vi "S2C_Access_ReadSettings.vi"(8 "Error In":errorcluster) -> (0 "Error Out":errorcluster)   [LabVIEW 2015]
doc: "Reads the data contained within the Settings file and loads the data into VI specific global variables."
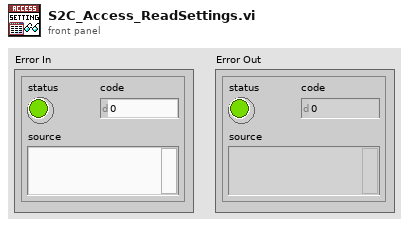
[diagram p1: front panel]
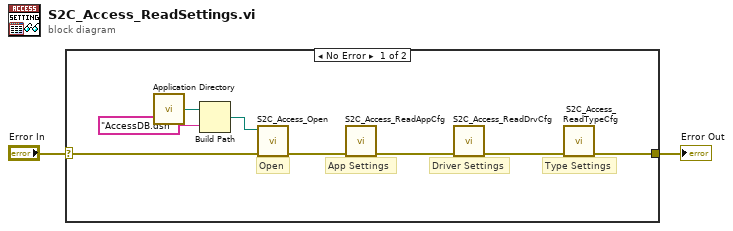
[diagram p0: block diagram]
diagram:
  n1 = case shown="No Error" "Error In" {
    selector: "Error In" -> [w10 w11]
    tunnel: [w6 w11] -> w1
    frame No Error {
      # "Type Settings"
      # "Driver Settings"
      # "App Settings"
      # "Open"
      n2 = call <vilib>:"Application Directory.vi"() -> ("Application Directory"=w4:path)
      n3 = Build Path(base path=w4, name or relative path="AccessDB.dsn") -> (appended path=w3:path)
      n4 = call "S2C_Access_Open.vi"("Error In"=w10, "DSN_Path"=w3) -> ("Error Out"=w9:errorcluster)  [unwired: 8 in, 1 out]
      n5 = call "S2C_Access_ReadAppCfg.vi"("Error In"=w9) -> ("Error Out"=w8:errorcluster)  [unwired: 10 in]
      n6 = call "S2C_Access_ReadDrvCfg.vi"("Error In"=w8) -> ("Error Out"=w7:errorcluster)  [unwired: 10 in]
      n7 = call "S2C_Access_ReadTypeCfg.vi"("Error In"=w7) -> ("Error Out"=w6:errorcluster)  [unwired: 10 in]
    }
    frame Error {
    }
  }
  "Error Out" <- w1
